vi "InsertCell.vi"(6 "Number":i32, 9 "Current Cell":T1, 11 "Board":i32[][](array[numeric])) -> (3 "Board":i32[][](array[numeric]))   [LabVIEW 2023]
doc: "Insert Number in Current Cell\n\nInputs\n- Board: Current Board Configuration\n- Row: Row of current Cell\n- Column: Column of current Cell\n- Number: Number to try out in current Cell\n\nOutputs\n- Board: Current Board Configuration\n- Row: Row of current Cell\n- Column: Column of current Cell"
uses:
  Controls/CurrentCell.ctl
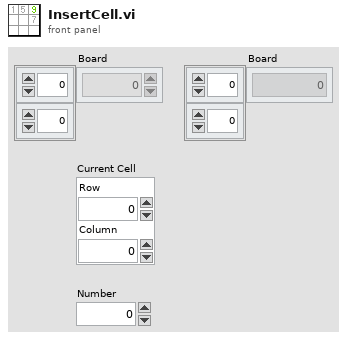
[diagram p1: front panel]
types:
  T1 = typedef "CurrentCell.ctl" = cluster{"Row":i32, "Column":i32}
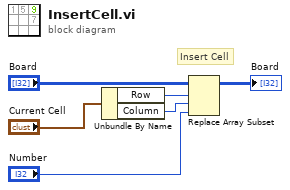
[diagram p0: block diagram]
diagram:
  # "Insert Cell"
  n1 = Unbundle By Name("Current Cell") -> ("Row"=w3:i32, "Column"=w2:i32)
  n2 = Replace Array Subset(array="Board", new element="Number", index (row)=w3, index (col)=w2) -> (→"Board":i32[][])
